vi "Inward_Lens_Tuning(GUI).vi"() -> ()   [LabVIEW 2019]
uses:
  Control/QMH Fundamentals - Message Cluster.ctl
panel:
  out "OUTWARD FOCUSING 3 RECHECK":bool
  out "OUTWARD FOCUSING 3 RECHECK":bool
  out "INWARD 2FOCUSING RECHECK":bool
  out "INWARD 1 FOCUSING  3 RECHECK":bool
  out "OUTWARD FOCUSING 2":bool
  out "OUTWARD FOCUSING 1":bool
  out "INWARD 2FOCUSING":bool
  out "INWARD 1 FOCUSING 2":bool
  in  "Project-Name 3":string="LensTuning"
  in  "Project-Name 2":string="LensTuning"
  in  "error in (no error)":errorcluster
  in  "Waveform Chart":refnum<vi>
  out "Result":bool=TRUE caption="RESULT"
  out "Progress Squence":bool=TRUE
  in  "Project-Name":string="LensTuning"
  in  "Test Start":bool
  in  "Test Stop":bool
  in  "Reset Counter":bool
  out "COUNTER":i32=66
  in  "SERIAL NUMBER":string="123A1C85540"
  out "TIME":string="02:37"
  out "DATE":string="25-08-2021"
  in  "Acquired Image":T1(plugin-control)
  in  "Stop Button":bool
  # "LENS TUNING STATION"
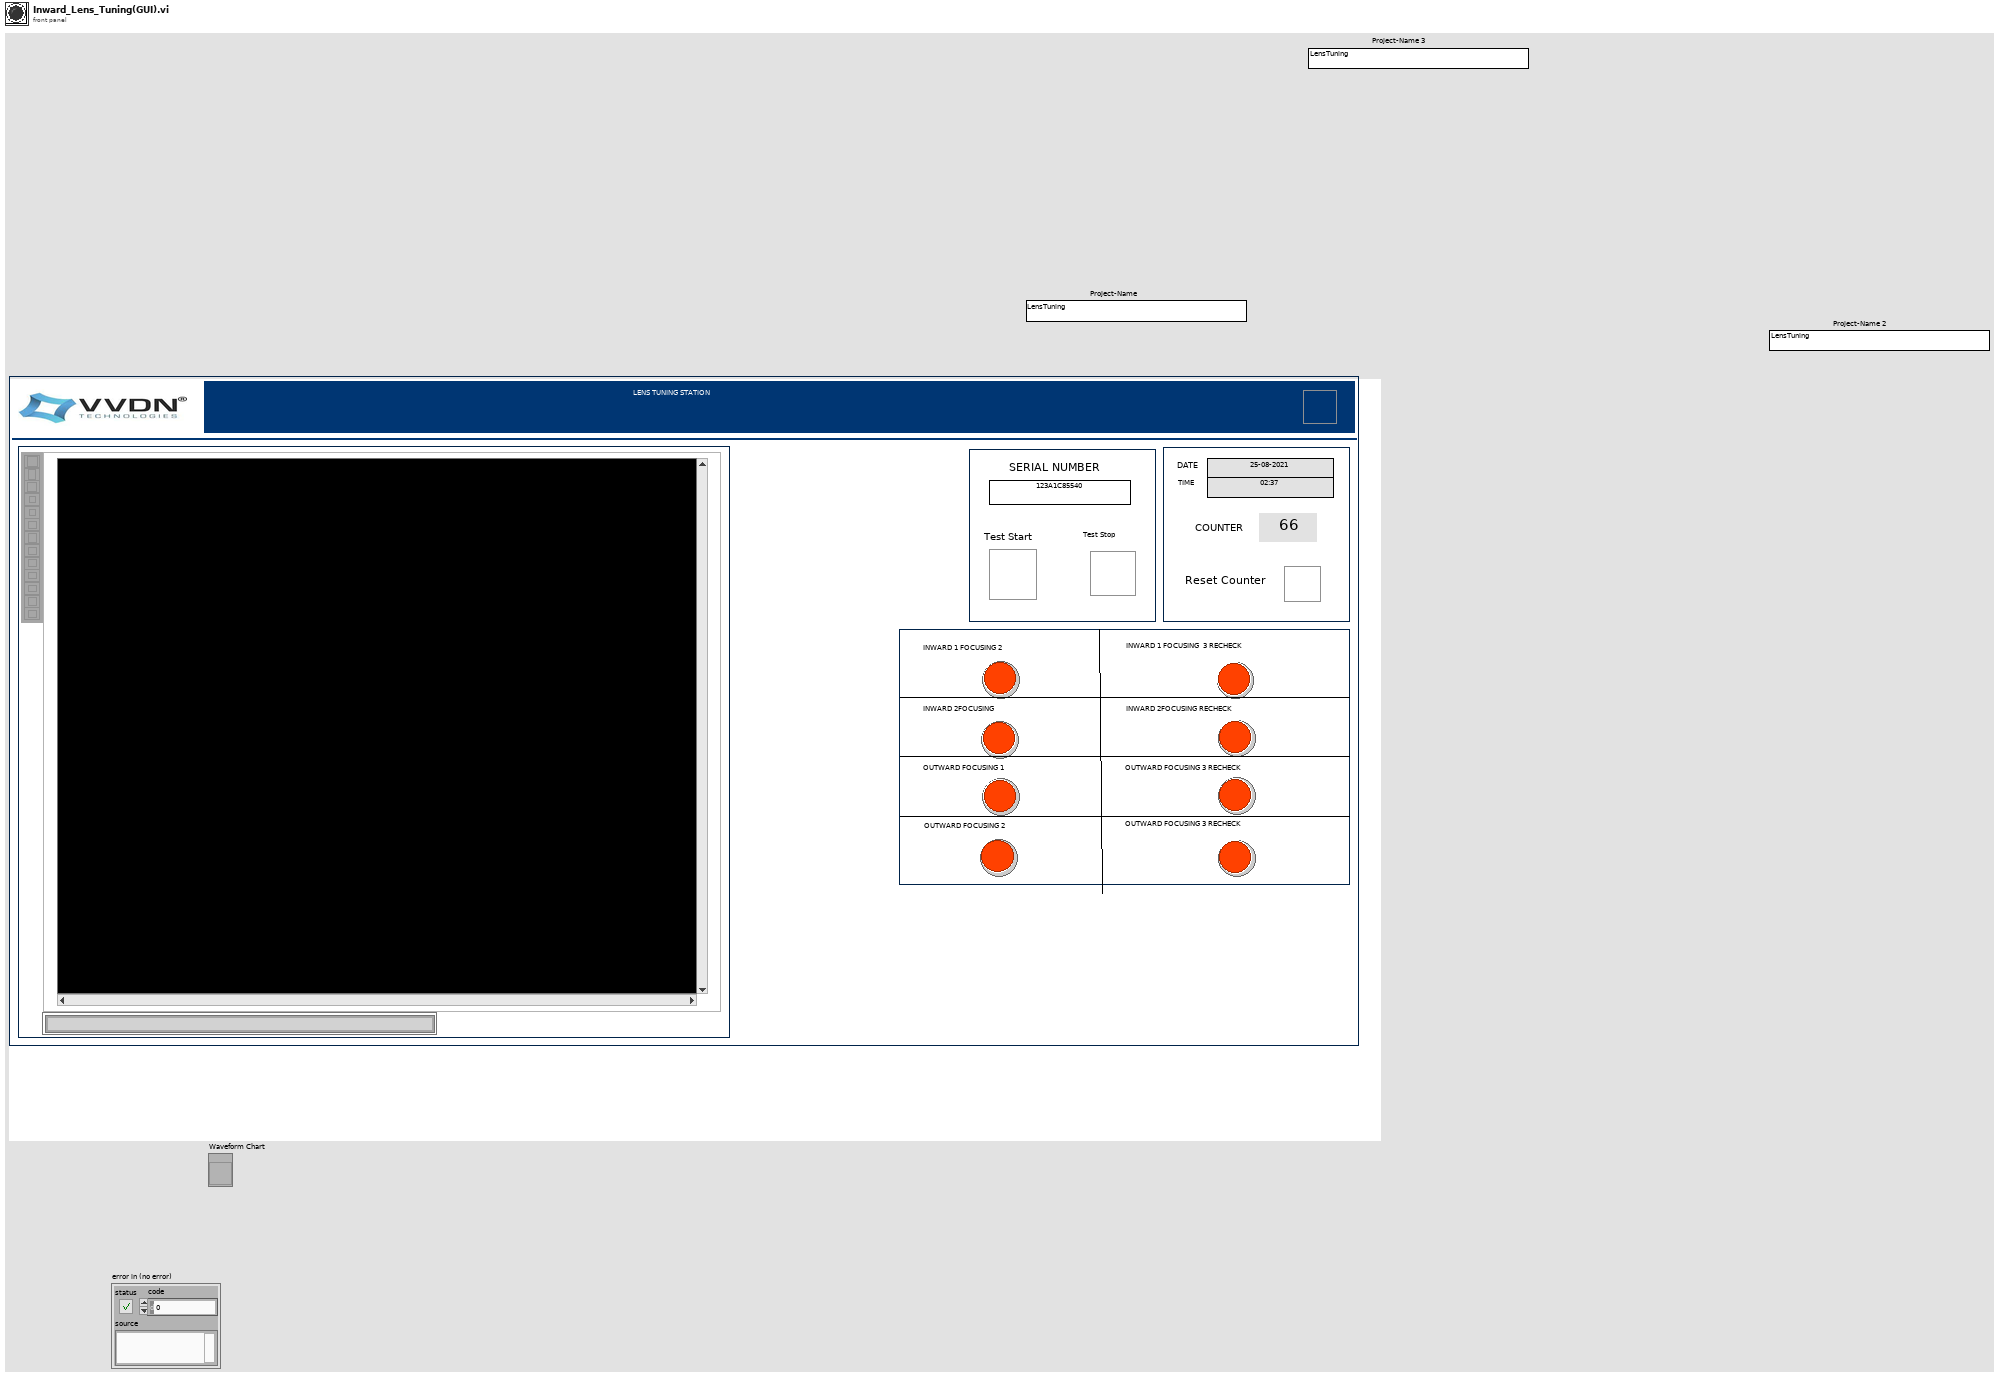
[diagram p1: front panel]
types:
  T1 = typedef "IMAQ Image.ctl" = refnum<image>
  T2 = typedef "QMH Fundamentals - Message Cluster.ctl" = cluster{"Message":string, "Message Data":variant}
  T3 = cluster{"RH_BOTTOM":bool, "RH_CENTER":bool, "RH_TOP":bool, "BOTTOM":bool, "CENTER":bool, "TOP":bool, "RH_BOTTOM   2":string, "RH_CENTER  2":string, "RH_TOP  2":string, "C_BOTTOM ":string, "C_CENTER 2":string, "C_TOP":string}
  T4 = enum32{"Invalid", "Standard", "Closed", "Hidden", "Minimized", "Maximized"}
  T5 = cluster{"C_Center":string, "Center 2":bool, "C_Top":string, "Top 2":bool, "C_Bottom":string, "Bottom 2":bool, "RH_TOP":string, "Top_RH":bool, "RH_CENTER":string, "Center_RH":bool, "RH_BOTTOM":string, "Bottom_RH":bool}
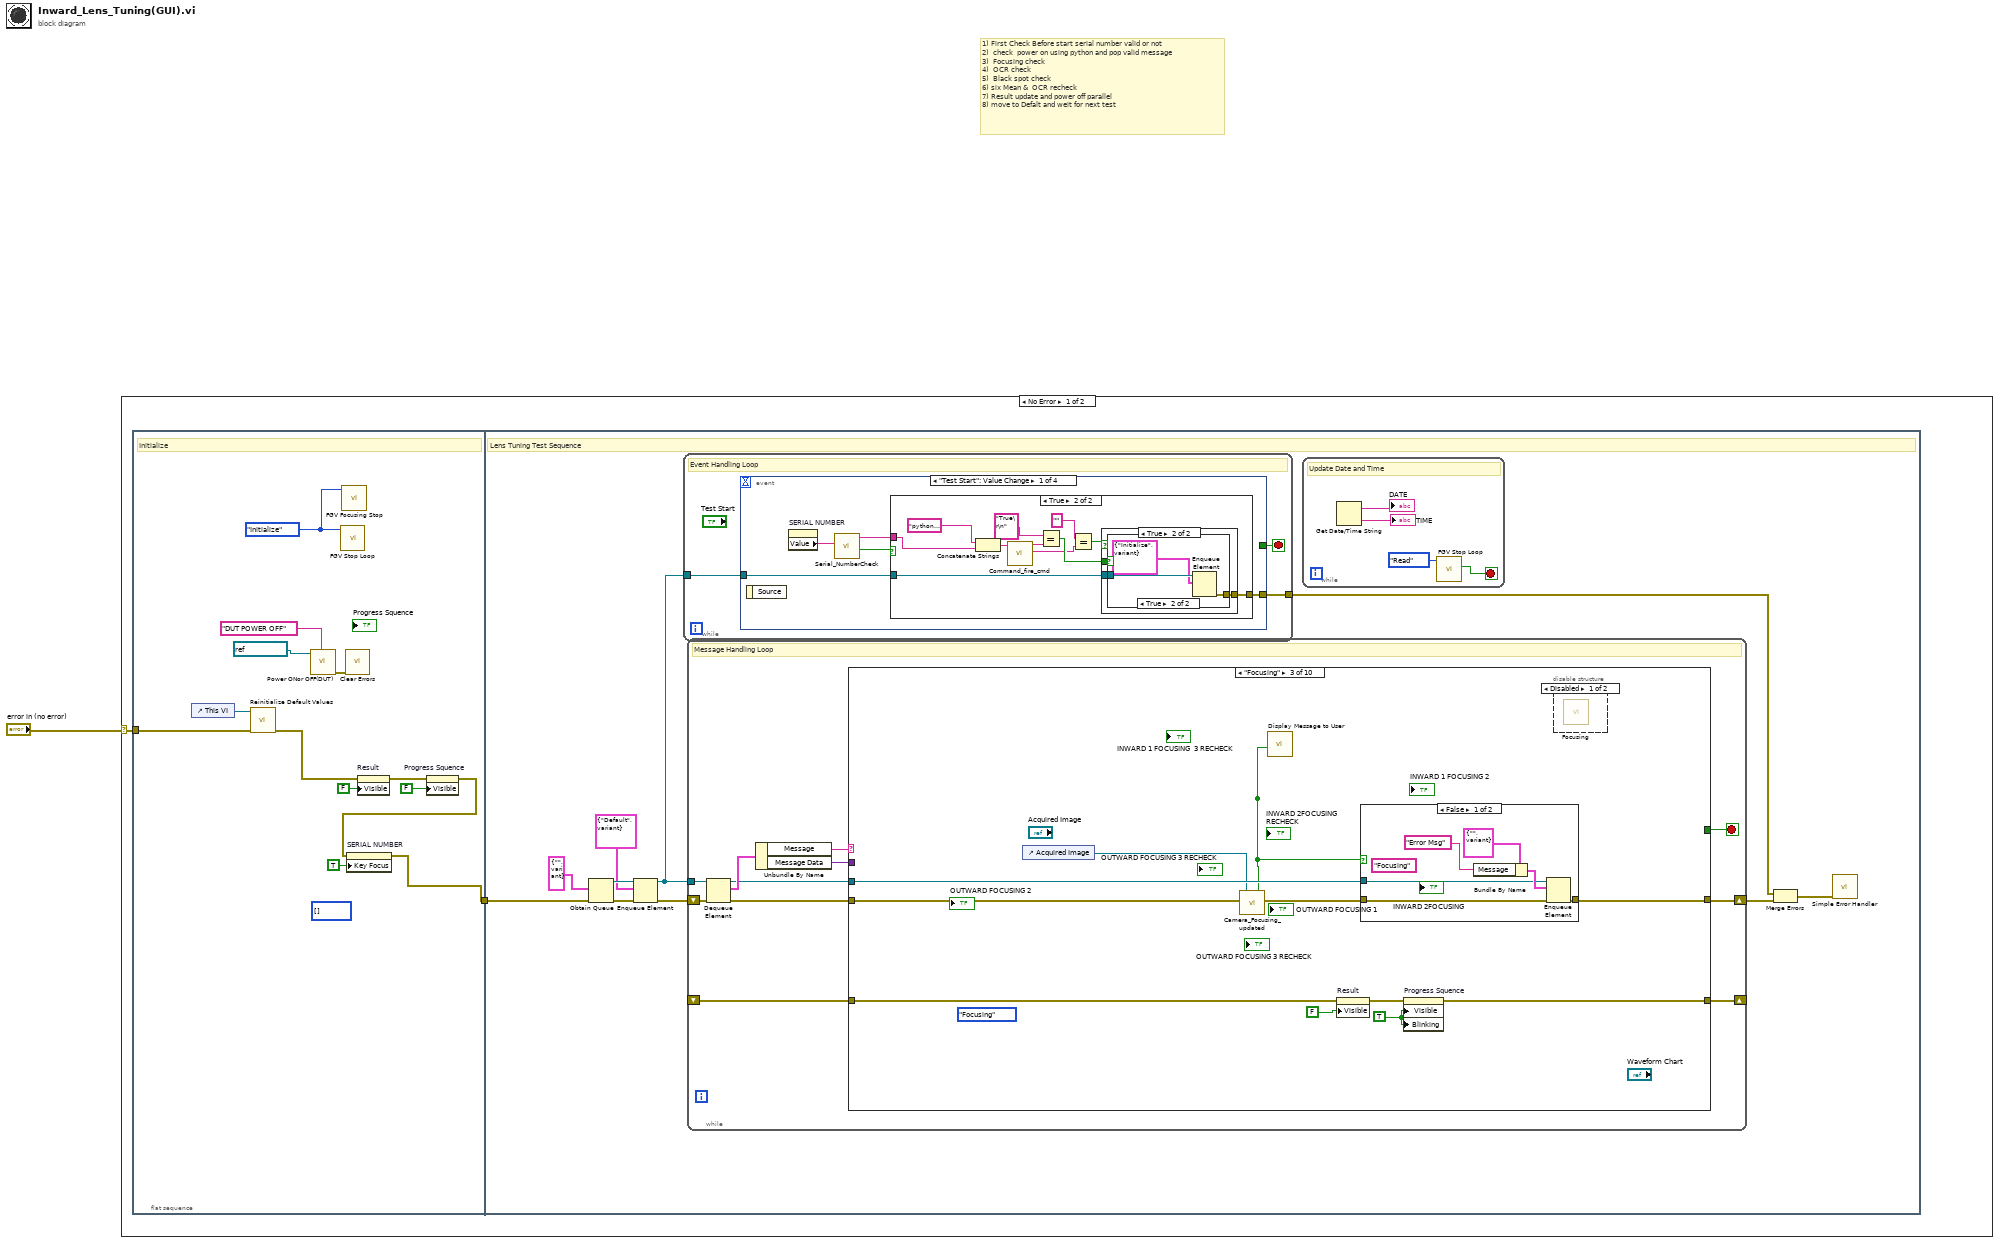
[diagram p0: block diagram]
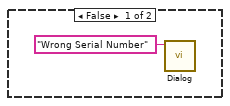
[diagram p2: hidden frame]
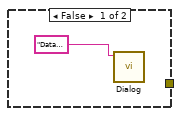
[diagram p3: hidden frame]
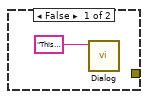
[diagram p4: hidden frame]
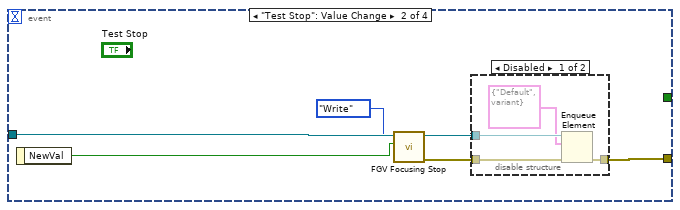
[diagram p5: hidden frame]
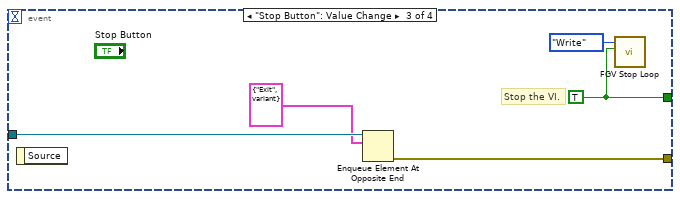
[diagram p7: hidden frame]
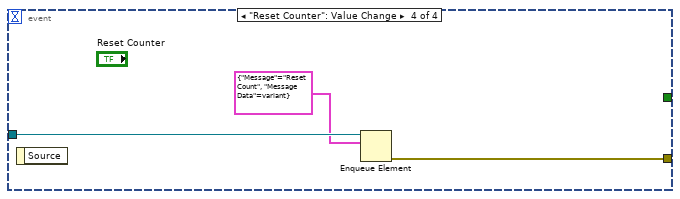
[diagram p8: hidden frame]
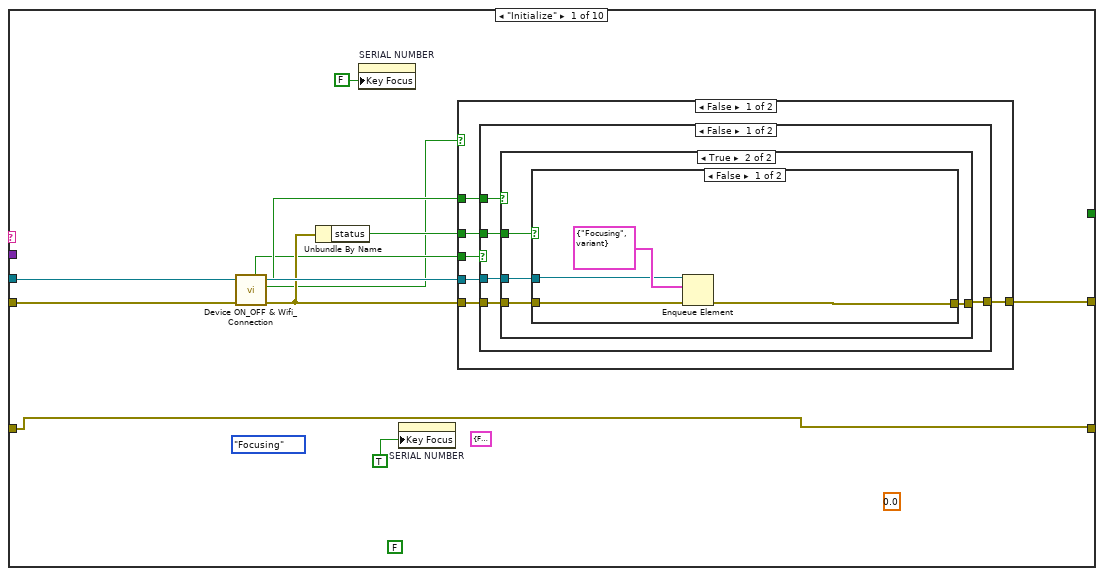
[diagram p9: hidden frame]
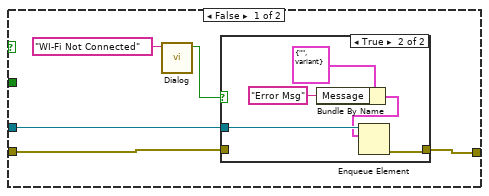
[diagram p10: hidden frame]
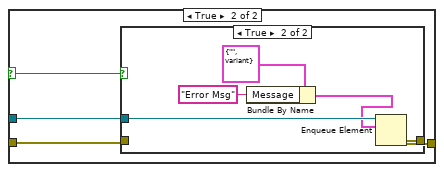
[diagram p12: hidden frame]
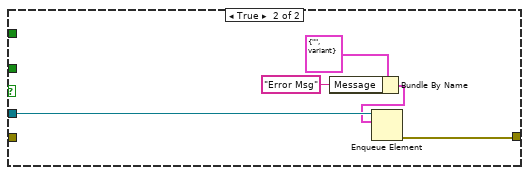
[diagram p14: hidden frame]
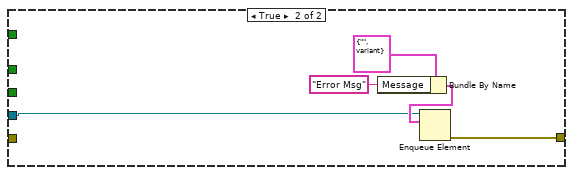
[diagram p15: hidden frame]
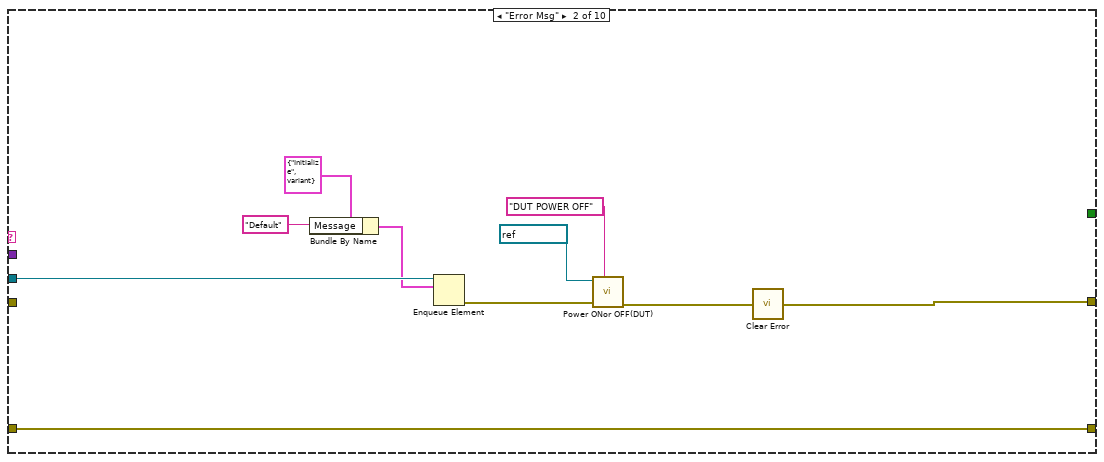
[diagram p16: hidden frame]
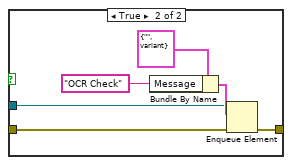
[diagram p18: hidden frame]
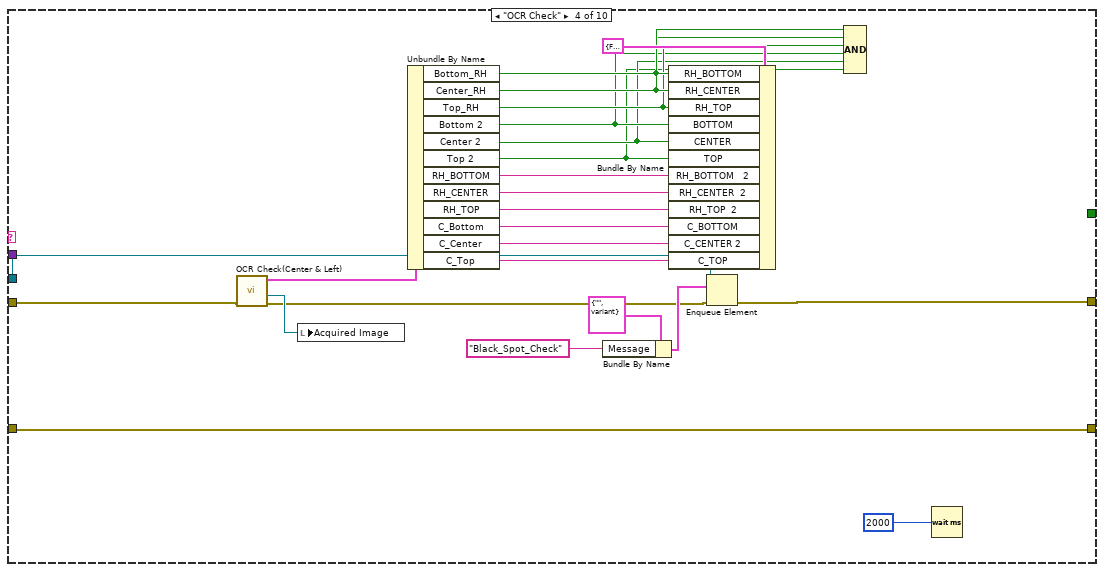
[diagram p19: hidden frame]
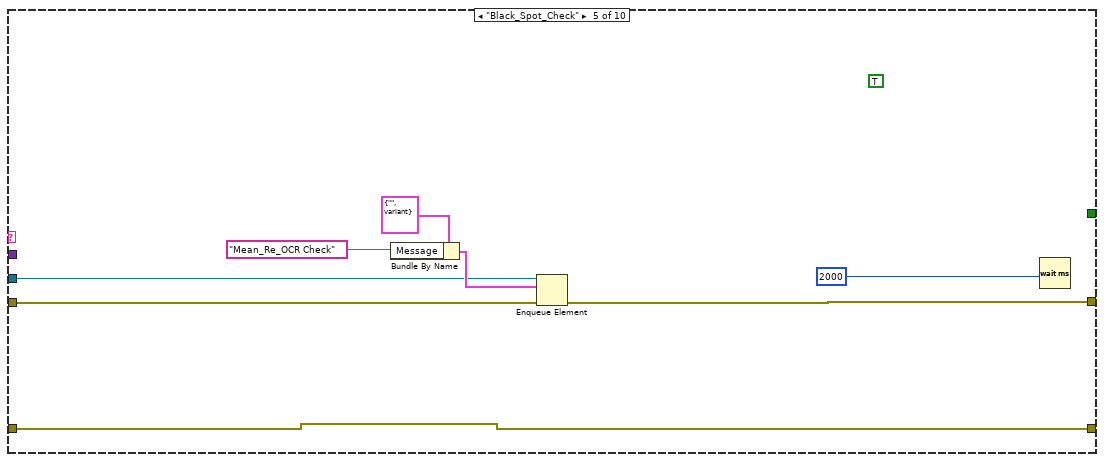
[diagram p20: hidden frame]
diagram:
  # "1) First Check Before start serial number valid or not\n2)  check  power on using python and pop valid message \n3)  Focusing check \n4)  OCR check\n5)  Black spot check\n6) six Mean &  OCR recheck\n7) Result update and power off parallel\n8) move to Defalt and weit for next test"
  n1 = case shown="No Error" "error in (no error)" {
    selector: "error in (no error)" -> [w2 _]
    frame No Error {
      n2 = flat-sequence {
        tunnel: [w4] -> w3
        tunnel: w2 -> [w10]
        tunnel: w3 -> [w18]
        frame #0 {
          (unwired) i32[] []
          w8 = enum16{"Initialize", "Read", "Write"}."Initialize" ("Action")
          # "Initialize"
          n3 = control-ref of="This VI"() -> (w13:refnum<vi>)
          n4 = call "Reinitialize Default Values.vi"("error in (no error)"=w10, "VI in"=w13) -> ("error out"=w9:errorcluster)  [unwired: 9 in]
          n5 = call "Power ONor OFF(DUT).vi"("String"="DUT POWER OFF", "VISA resource name"=refnum<visa-resource-name> "COM11") -> ("error out"=w5:errorcluster)  [unwired: 9 in]
          n6 = call "FGV Stop Loop.vi"("Action"=w8) -> ()  [unwired: 9 in, 2 out]
          n7 = call "FGV Focusing Stop.vi"("Action"=w8) -> ()  [unwired: 9 in, 2 out]
          n8 = call <vilib>:"Clear Errors.vi"("error in (no error)"=w5) -> ()  [unwired: 5 in, 2 out]
          n9 = property on="Result" class="Bool (strict)"(error in=w9, "Visible"=FALSE) -> (error out=w16:errorcluster)  [unwired: 1 in, 1 out]
          n10 = property on="Progress Squence" class="Bool (strict)"(error in=w16, "Visible"=FALSE) -> (error out=w12:errorcluster)  [unwired: 1 in, 1 out]
          n11 = property on="SERIAL NUMBER" class="Str"(error in=w12, "Key Focus"=TRUE) -> (error out=w4:errorcluster)  [unwired: 1 in, 1 out]
        }
        frame #1 {
          # "Lens Tuning Test Sequence"
          n12 = Obtain Queue(element data type=T2 {"Message"="", "Message Data"=variant} ("Message Cluster"), error in (no error)=w18) -> (queue out=w23:refnum<queue>, error out=w24:errorcluster)  [unwired: 3 in, 1 out]
          n13 = Enqueue Element(queue=w23, element=T2 {"Message"="Default", "Message Data"=variant}, error in (no error)=w24) -> (queue out=w21:refnum<queue>, error out=w22:errorcluster)  [unwired: 1 in, 1 out]
          n14 = while {
            tunnel: w21 -> [w33]
            tunnel: [w31] -> w26
            stop <- w32 stop-if-true
            # "Event Handling Loop"
            n15 = event shown="[0] \"Test Start\": Value Change" {
              selector: _ -> [_ _ _ _]
              dyn-events: _ -> [_ _ _ _]
              timeout: _ -> [_ _ _ _]
              tunnel: [_ _ w68 _] -> w32
              tunnel: w33 -> [w38 w63 w72 w75]
              tunnel: [w37 w62 w71 w74] -> w31
              event "Test Start": Value Change {
                n16 = event-data() -> ()  [unwired: 1 in, 1 out]
                n17 = property on="SERIAL NUMBER" class="Str"() -> ("Value"=w35:string)  [unwired: 2 in, 2 out]
                n18 = call "Serial_NumberCheck.vi"("Serial Number In"=w35) -> ("Serial Number"=w36:bool, "Serial number out"=w34:string)  [unwired: 9 in]
                n19 = case shown="True" w36 {
                  tunnel: w38 -> [_ w50]
                  tunnel: [_ w49] -> w37
                  tunnel: w34 -> [_ w45]
                  frame False {
                    n20 = call "Dialog.vi"("Status"="Wrong Serial Number") -> ()  [unwired: 10 in, 1 out]
                  }
                  frame True {
                    n21 = Concatenate Strings("python C:\\\\Users\\\\vvdn\\\\Downloads\\\\check_upd_db.py ", w45) -> (w48:string)
                    n22 = call "Command_fire_cmd.vi"("command line"=w48) -> ("standard error"=w40:string, "standard output"=w47:string)  [unwired: 6 in, 1 out]
                    n23 = Equal?(x="True\r\n" ("standard output"), y=w47) -> (x = y?=w43:bool)
                    n24 = Equal?(x="" ("standard error"), y=w40) -> (x = y?=w41:bool)
                    n25 = case shown="True" w41 {
                      tunnel: w50 -> [_ w54]
                      tunnel: [_ w53] -> w49
                      tunnel: w43 -> [_ w52]
                      frame False {
                        n26 = call "Dialog.vi"("Status"="Database Connection Error ") -> ()  [unwired: 10 in, 1 out]
                      }
                      frame True {
                        n27 = case shown="True" w52 {
                          tunnel: w54 -> [_ w58]
                          tunnel: [_ w57] -> w53
                          frame False {
                            n28 = call "Dialog.vi"("Status"="This Serial Number Not Exist in Database  ") -> ()  [unwired: 10 in, 1 out]
                          }
                          frame True {
                            n29 = Enqueue Element(queue=w58, element=T2 {"Message"="Initialize", "Message Data"=variant}) -> (error out=w57:errorcluster)  [unwired: 2 in, 2 out]
                          }
                        }
                      }
                    }
                  }
                }
              }
              event "Test Stop": Value Change {
                n30 = event-data() -> ("NewVal"=w60:bool)  [unwired: 1 in]
                n31 = call "FGV Focusing Stop.vi"("In"=w60, "Action"=enum16{"Initialize", "Read", "Write"}."Write") -> ("error out"=w59:errorcluster)  [unwired: 8 in, 1 out]
                n32 = disable-structure shown="Disabled" {
                  disable-tunnel: w63 -> [w67 _]
                  disable-tunnel: [w66 _] -> w62
                  disable-tunnel: w59 -> [w64 _]
                  frame Disabled {
                    n33 = Enqueue Element(queue=w67, element=T2 {"Message"="Default", "Message Data"=variant}, error in (no error)=w64) -> (error out=w66:errorcluster)  [unwired: 1 in, 2 out]
                  }
                  frame Enabled {
                  }
                }
              }
              event "Stop Button": Value Change {
                w68 = TRUE
                # "Stop the VI."
                n34 = event-data() -> ()  [unwired: 1 in, 1 out]
                n35 = Enqueue Element At Opposite End(queue=w72, element=T2 {"Message"="Exit", "Message Data"=variant}) -> (error out=w71:errorcluster)  [unwired: 2 in, 2 out]
                n36 = call "FGV Stop Loop.vi"("In"=w68, "Action"=enum16{"Initialize", "Read", "Write"}."Write") -> ()  [unwired: 8 in, 2 out]
              }
              event "Reset Counter": Value Change {
                n37 = event-data() -> ()  [unwired: 1 in, 1 out]
                n38 = Enqueue Element(queue=w75, element=T2 {"Message"="Reset Count", "Message Data"=variant}) -> (error out=w74:errorcluster)  [unwired: 2 in, 2 out]
              }
            }
          }
          n39 = while {
            tunnel: w21 -> [w84]
            shift-right: [w78] -> _
            shift-left: _ -> [w77]
            shift-right: [w76] -> w17
            shift-left: w22 -> [w85]
            stop <- w86 stop-if-true
            # "Message Handling Loop"
            n40 = Dequeue Element(queue=w84, error in (no error)=w85) -> (queue out=w82:refnum<queue>, element=w83:T2, error out=w81:errorcluster)  [unwired: 1 in, 1 out]
            n41 = Unbundle By Name(w83) -> ("Message"=w80:string, "Message Data"=w79:variant)
            n42 = case "Message Cases" shown="\"Focusing\"" w80 {
              tunnel: w82 -> [w99 w158 w171 w210 w216 w230 w265 w283 w295 _]
              tunnel: w81 -> [w93 _ w163 w189 w215 w222 w251 w282 w293 w313]
              tunnel: [w94 w150 w170 w209 w214 w228 w264 w281 w288 w316] -> w76
              tunnel: [_ _ _ _ _ _ _ _ TRUE _] -> w86
              tunnel: w79 -> [_ _ _ _ _ _ _ _ _ _]
              tunnel: [w88 w159 w164 w186 w211 w220 w252 w271 w287 w297] -> w78
              tunnel: w77 -> [w88 w159 w160 w186 w211 w220 w233 w271 w287 w298]
              frame "Initialize" {
                (unwired) T3 {"RH_BOTTOM"=FALSE, "RH_CENTER"=FALSE, "RH_TOP"=FALSE, "BOTTOM"=FALSE, "CENTER"=FALSE, "TOP"=FALSE, "RH_BOTTOM   2"="", "RH_CENTER  2"="", "RH_TOP  2"="", "C_BOTTOM "="", "C_CENTER 2"="", "C_TOP"=""} ("OCR Check")
                w96 = 0.0 ("MEAN VALUE MAX")
                w95 = FALSE ("OCR CHECK")
                (unwired) enum32{"Focusing", "OCR Check"}."Focusing" ("Tab Control")
                # "Initialize - Perform any initialization code for your application here. In this example, the only initialization required is setting the Display Message indicator value to an empty string."
                n43 = call "Device ON_OFF & Wifi_Connection.vi"("error in"=w93) -> ("error out"=w92:errorcluster, "DUT COM port"=w89:bool, "Wifi Connected"=w91:bool, "Device Not respond"=w90:bool)  [unwired: 7 in]
                n44 = Unbundle By Name(w92) -> ("status"=w97:bool)
                n45 = property on="SERIAL NUMBER" class="Str"("Key Focus"=FALSE) -> ()  [unwired: 2 in, 2 out]
                n46 = property on="SERIAL NUMBER" class="Str"("Key Focus"=TRUE) -> ()  [unwired: 2 in, 2 out]
                n47 = case shown="False" w89 {
                  tunnel: w99 -> [w105 w145]
                  tunnel: w97 -> [w104 _]
                  tunnel: [w103 w146] -> w94
                  tunnel: w92 -> [w102 _]
                  tunnel: w91 -> [w101 _]
                  tunnel: w90 -> [w100 _]
                  frame False {
                    n48 = case shown="False" w100 {
                      tunnel: w105 -> [w110 w142]
                      tunnel: w104 -> [w109 _]
                      tunnel: [w108 w141] -> w103
                      tunnel: w102 -> [w107 _]
                      tunnel: w101 -> [w106 _]
                      frame False {
                        n49 = case shown="True" w106 {
                          tunnel: w107 -> [w113 w125]
                          tunnel: w110 -> [w114 w124]
                          tunnel: [w112 w123] -> w108
                          tunnel: w109 -> [_ w122]
                          frame False {
                            n50 = call "Dialog.vi"("Status"="WI-Fi Not Connected") -> ("Cancelled?"=w111:bool)  [unwired: 10 in]
                            n51 = case shown="True" w111 {
                              tunnel: w114 -> [_ w121]
                              tunnel: w113 -> [w116 _]
                              tunnel: [w116 w120] -> w112
                              frame False {
                              }
                              frame True {
                                n52 = Bundle By Name(cluster=T2 {"Message"="", "Message Data"=variant} ("Message Cluster"), "Message"="Error Msg") -> (w118:T2)
                                n53 = Enqueue Element(queue=w121, element=w118) -> (error out=w120:errorcluster)  [unwired: 2 in, 2 out]
                              }
                            }
                          }
                          frame True {
                            n54 = case shown="False" w122 {
                              selector: w122 -> [_ w130]
                              tunnel: w125 -> [w127 w132]
                              tunnel: w124 -> [w128 w133]
                              tunnel: [w126 w131] -> w123
                              frame False {
                                n55 = Enqueue Element(queue=w128, element=T2 {"Message"="Focusing", "Message Data"=variant}, error in (no error)=w127) -> (error out=w126:errorcluster)  [unwired: 1 in, 2 out]
                              }
                              frame True {
                                n56 = case shown="True" w130 {
                                tunnel: w133 -> [_ w139]
                                tunnel: w132 -> [w134 _]
                                tunnel: [w134 w138] -> w131
                                frame False {
                                }
                                frame True {
                                n57 = Bundle By Name(cluster=T2 {"Message"="", "Message Data"=variant} ("Message Cluster"), "Message"="Error Msg") -> (w136:T2)
                                n58 = Enqueue Element(queue=w139, element=w136) -> (error out=w138:errorcluster)  [unwired: 2 in, 2 out]
                                }
                                }
                              }
                            }
                          }
                        }
                      }
                      frame True {
                        n59 = Bundle By Name(cluster=T2 {"Message"="", "Message Data"=variant} ("Message Cluster"), "Message"="Error Msg") -> (w140:T2)
                        n60 = Enqueue Element(queue=w142, element=w140) -> (error out=w141:errorcluster)  [unwired: 2 in, 2 out]
                      }
                    }
                  }
                  frame True {
                    n61 = Bundle By Name(cluster=T2 {"Message"="", "Message Data"=variant} ("Message Cluster"), "Message"="Error Msg") -> (w149:T2)
                    n62 = Enqueue Element(queue=w145, element=w149) -> (error out=w146:errorcluster)  [unwired: 2 in, 2 out]
                  }
                }
              }
              frame "Error Msg" {
                n63 = Bundle By Name(cluster=T2 {"Message"="Initialize", "Message Data"=variant} ("element"), "Message"="Default") -> (w155:T2)
                n64 = Enqueue Element(queue=w158, element=w155) -> (error out=w152:errorcluster)  [unwired: 2 in, 2 out]
                n65 = call "Power ONor OFF(DUT).vi"("String"="DUT POWER OFF", "error in (no error)"=w152, "VISA resource name"=refnum<visa-resource-name> "COM11") -> ("error out"=w151:errorcluster)  [unwired: 8 in]
                n66 = call "Clear Error.vi"("error in"=w151) -> ("error out"=w150:errorcluster)
              }
              frame "Focusing" {
                w173 = TRUE ("Visible")
                (unwired) enum32{"Focusing", "OCR Check"}."Focusing" ("Tab Control")
                n67 = control-ref of="Acquired Image"() -> (w167:refnum<vi>)
                n68 = call "Camera_Focusing_updated.vi"("error in"=w163, "Ctl Refnum"=w167) -> ("CURRENT MEAN VALUE"=w169:refnum<vi>, "MEAN VALUE MAX"=w168:refnum<vi>, "Result"=w161:bool, "Pattern Presence"=w166:refnum<vi>, "error out"=w162:errorcluster)  [unwired: 8 in, 5 out]
                n69 = call "Display Message to User"("Enable"=w161) -> ()  [unwired: 9 in, 2 out]
                n70 = property on="Result" class="Bool (strict)"(error in=w160, "Visible"=FALSE) -> (error out=w165:errorcluster)  [unwired: 1 in, 1 out]
                n71 = case shown="False" w161 {
                  tunnel: w171 -> [w176 w182]
                  tunnel: w162 -> [w177 w181]
                  tunnel: [w175 w180] -> w170
                  frame False {
                    (unwired) "Focusing" ("Message")
                    n72 = Bundle By Name(cluster=T2 {"Message"="", "Message Data"=variant} ("Message Cluster"), "Message"="Error Msg") -> (w179:T2)
                    n73 = Enqueue Element(queue=w176, element=w179, error in (no error)=w177) -> (error out=w175:errorcluster)  [unwired: 1 in, 2 out]
                  }
                  frame True {
                    n74 = Bundle By Name(cluster=T2 {"Message"="", "Message Data"=variant} ("Message Cluster"), "Message"="OCR Check") -> (w185:T2)
                    n75 = Enqueue Element(queue=w182, element=w185, error in (no error)=w181) -> (error out=w180:errorcluster)  [unwired: 1 in, 2 out]
                  }
                }
                n76 = property on="Progress Squence" class="Bool (strict)"(error in=w165, "Visible"=w173, "Blinking"=w173) -> (error out=w164:errorcluster)  [unwired: 1 in, 1 out]
                n77 = disable-structure shown="Disabled" {
                  frame Disabled {
                    n78 = call "Focusing.vi"() -> ()  [unwired: 7 in, 5 out]
                  }
                  frame Enabled {
                  }
                }
              }
              frame "OCR Check" {
                n79 = call "OCR Check(Center & Left).vi"("error in (no error)"=w189) -> ("error out"=w188:errorcluster, "Image Out"=w190:T1, "RIGHT"=w187:bool, "OCR Check"=w206:T5)  [unwired: 6 in, 1 out]
                n80 = local write "Acquired Image"(w190) -> ()
                n81 = Unbundle By Name(w206) -> ("Bottom_RH"=w199:bool, "Center_RH"=w198:bool, "Top_RH"=w197:bool, "Bottom 2"=w196:bool, "Center 2"=w195:bool, "Top 2"=w194:bool, "RH_BOTTOM"=w200:string, "RH_CENTER"=w201:string, "RH_TOP"=w202:string, "C_Bottom"=w203:string, "C_Center"=w204:string, "C_Top"=w205:string)
                n82 = Bundle By Name(cluster=T2 {"Message"="", "Message Data"=variant} ("Message Cluster"), "Message"="Black_Spot_Check") -> (w191:T2)
                n83 = Bundle By Name(cluster=T3 {"RH_BOTTOM"=FALSE, "RH_CENTER"=FALSE, "RH_TOP"=FALSE, "BOTTOM"=FALSE, "CENTER"=FALSE, "TOP"=FALSE, "RH_BOTTOM   2"="", "RH_CENTER  2"="", "RH_TOP  2"="", "C_BOTTOM "="", "C_CENTER 2"="", "C_TOP"=""} ("OCR Check"), "RH_BOTTOM"=w199, "RH_CENTER"=w198, "RH_TOP"=w197, "BOTTOM"=w196, "CENTER"=w195, "TOP"=w194, "RH_BOTTOM   2"=w200, "RH_CENTER  2"=w201, "RH_TOP  2"=w202, "C_BOTTOM"=w203, "C_CENTER 2"=w204, "C_TOP"=w205) -> ()  [unwired: 1 out]
                n84 = Enqueue Element(queue=w210, element=w191, error in (no error)=w188) -> (error out=w209:errorcluster)  [unwired: 1 in, 2 out]
                n85 = Compound Arithmetic op=AND(w199, w198, w197, w196, w195, w194) -> ()  [unwired: 1 out]
                n86 = Wait (ms)(milliseconds to wait=u32 2000) -> ()  [unwired: 1 out]
              }
              frame "Black_Spot_Check" {
                w213 = TRUE ("BLACK SPOT CHECK")
                # "Update Display - Convert the Message Data to a string to display in the Display Message indicator."
                n87 = Bundle By Name(cluster=T2 {"Message"="", "Message Data"=variant} ("Message Cluster"), "Message"="Mean_Re_OCR Check") -> (w219:T2)
                n88 = Enqueue Element(queue=w216, element=w219, error in (no error)=w215) -> (error out=w214:errorcluster)  [unwired: 1 in, 2 out]
                n89 = Wait (ms)(milliseconds to wait=u32 2000) -> ()  [unwired: 1 out]
              }
              frame "Mean_Re_OCR Check" {
                (unwired) TRUE ("MEAN & REOCR CHECK")
                n90 = control-ref of="Acquired Image"() -> (w226:refnum<vi>)
                n91 = call "Camera_Mean_OCR_recheck.vi"("Ctl Refnum"=w226, "error in (no error)"=w222) -> ("OCR Recheck"=w223:bool, "Mean Value Max"=w225:sgl, "Curent Mean Value"=w224:sgl, "error out"=w221:errorcluster)  [unwired: 7 in, 3 out]
                n92 = Bundle By Name(cluster=T2 {"Message"="", "Message Data"=variant} ("Message Cluster"), "Message"="Result Update") -> (w229:T2)
                n93 = Enqueue Element(queue=w230, element=w229, error in (no error)=w221) -> (error out=w228:errorcluster)  [unwired: 1 in, 2 out]
                n94 = Wait (ms)(milliseconds to wait=u32 2000) -> ()  [unwired: 1 out]
              }
              frame "Result Update" {
                w256 = FALSE ("Visible")
                n95 = Compound Arithmetic op=AND() -> (w257:bool, w263:bool, w262:bool, w261:bool, w260:bool)
                "Result" <- w257
                n96 = Build Array(w263, w262, w261, w260, w257) -> (w258:bool[])
                n97 = call "Reports.vi"("SERIAL NUMBER"="SERIAL NUMBER", "Result"=w258, "error in"=w251) -> ("error out"=w248:errorcluster)  [unwired: 6 in]
                n98 = property on="Progress Squence" class="Bool (strict)"(error in=w233, "Visible"=w256, "Blinking"=w256) -> (error out=w253:errorcluster)  [unwired: 1 in, 1 out]
                n99 = call "Power ONor OFF(DUT).vi"("String"="DUT POWER OFF", "error in (no error)"=w248, "VISA resource name"=refnum<visa-resource-name> "COM11") -> ("error out"=w247:errorcluster)  [unwired: 8 in]
                n100 = property on="Result" class="Bool (strict)"(error in=w253, "Visible"=TRUE) -> (error out=w252:errorcluster)  [unwired: 1 in, 1 out]
                n101 = call "Clear Error.vi"("error in"=w247) -> ("error out"=w246:errorcluster)
                n102 = Bundle By Name(cluster=T2 {"Message"="", "Message Data"=variant} ("Message Cluster"), "Message"="Default") -> (w267:T2)
                n103 = call <vilib>:"Application Directory.vi"() -> ("Application Directory"=w238:path)
                n104 = Enqueue Element(queue=w265, element=w267, error in (no error)=w246) -> (error out=w264:errorcluster)  [unwired: 1 in, 2 out]
                n105 = Build Path(base path=w238, name or relative path="VVDN") -> (appended path=w240:path)
                n106 = Concatenate Strings("Project-Name 3", "Counter.bin" ("string")) -> (w242:string)
                n107 = call "Check and Create Folder.vi"("Path In"=w240) -> ("error out"=w234:errorcluster, "Path Out"=w241:path)  [unwired: 8 in, 1 out]
                n108 = property on="COUNTER" class="DigNum (strict)"() -> ("Value"=w243:i32)  [unwired: 2 in, 2 out]
                n109 = Build Path(base path=w241, name or relative path=w242) -> (appended path=w235:path)
                n110 = Increment(x=w243) -> (x+1=w244:i32)
                n111 = call "Read&Write Counter.vi"("error in"=w234, "Count IN"=w244, "Path In"=w235) -> ("Count OUT"=→"COUNTER":i32)  [unwired: 7 in, 1 out]
                n112 = property on="SERIAL NUMBER" class="Str"("Key Focus"=TRUE) -> ()  [unwired: 2 in, 2 out]
              }
              frame "Reset Count" {
                n113 = Bundle By Name(cluster=T2 {"Message"="", "Message Data"=variant} ("Message Cluster"), "Message"="Default") -> (w285:T2)
                n114 = Enqueue Element(queue=w283, element=w285, error in (no error)=w282) -> (error out=w281:errorcluster)  [unwired: 1 in, 2 out]
                n115 = call <vilib>:"Application Directory.vi"() -> ("Application Directory"=w274:path)
                n116 = Build Path(base path=w274, name or relative path="VVDN") -> (appended path=w276:path)
                n117 = Concatenate Strings("Project-Name", "Counter.bin" ("string")) -> (w278:string)
                n118 = call "Check and Create Folder.vi"("Path In"=w276) -> ("error out"=w280:errorcluster, "Path Out"=w277:path)  [unwired: 8 in, 1 out]
                n119 = Build Path(base path=w277, name or relative path=w278) -> (appended path=w279:path)
                n120 = call "Read&Write Counter.vi"("error in"=w280, "Count IN"=0, "Path In"=w279) -> ("Count OUT"=w269:i32)  [unwired: 7 in, 1 out]
                n121 = property on="COUNTER" class="DigNum (strict)"("Value"=w269) -> ()  [unwired: 2 in, 2 out]
              }
              frame "Exit" {
                # "Stop the VI."
                # "Exit - Exit the application."
                n122 = Release Queue(queue=w295, error in (no error)=w293) -> (error out=w289:errorcluster)  [unwired: 1 in, 2 out]
                n123 = call "Open and Close-VI.vi"("State"=T4."Minimized", "Close VI"=path "Inward_Lens_Tuning(GUI).vi", "error in"=w289, "Open VI"=path "Lens_Tuning_Login.vi") -> ("error out"=w288:errorcluster)  [unwired: 11 in]
              }
              frame Default {
                w299 = FALSE ("Visible")
                n124 = property on="SERIAL NUMBER" class="Str"("Key Focus"=TRUE) -> ()  [unwired: 2 in, 2 out]
                n125 = call <vilib>:"Application Directory.vi"() -> ("Application Directory"=w305:path)
                n126 = Build Path(base path=w305, name or relative path="VVDN") -> (appended path=w307:path)
                n127 = Concatenate Strings("Project-Name 2", "Counter.bin" ("string")) -> (w309:string)
                n128 = call "Check and Create Folder.vi"("Path In"=w307) -> ("error out"=w311:errorcluster, "Path Out"=w308:path)  [unwired: 8 in, 1 out]
                n129 = property on="Progress Squence" class="Bool (strict)"(error in=w298, "Visible"=w299, "Blinking"=w299) -> (error out=w297:errorcluster)  [unwired: 1 in, 1 out]
                n130 = Build Path(base path=w308, name or relative path=w309) -> (appended path=w310:path)
                n131 = property on="SERIAL NUMBER" class="Str"(error in=w313, "Value"="") -> (error out=w314:errorcluster)  [unwired: 1 in, 1 out]
                n132 = call "Read&Write Counter.vi"("error in"=w311, "Count IN"=0, "Write/Read"=FALSE, "Path In"=w310) -> ("Count OUT"=w304:i32)  [unwired: 6 in, 1 out]
                n133 = property on="SERIAL NUMBER" class="Str"(error in=w314, "Key Focus"=TRUE) -> (error out=w316:errorcluster)  [unwired: 1 in, 1 out]
                n134 = property on="COUNTER" class="DigNum (strict)"("Value"=w304) -> ()  [unwired: 2 in, 2 out]
                n135 = call "FGV Focusing Stop.vi"("Action"=enum16{"Initialize", "Read", "Write"}."Initialize") -> ()  [unwired: 9 in, 2 out]
              }
            }
          }
          n136 = while {
            stop <- w28 stop-if-true
            # "Update Date and Time"
            n137 = Get Date/Time String() -> (date string=→"DATE":string, time string=→"TIME":string)  [unwired: 3 in]
            n138 = call "FGV Stop Loop.vi"("Action"=enum16{"Initialize", "Read", "Write"}."Read") -> ("Out"=w28:bool)  [unwired: 9 in, 1 out]
          }
          n139 = Merge Errors(w26, w17) -> (w19:errorcluster)
          n140 = call <vilib>:"Simple Error Handler.vi"("error in (no error)"=w19) -> ()  [unwired: 4 in, 5 out]
        }
      }
    }
    frame Error {
    }
  }
